vi "Synchronized PUT Channel.vi"(1 "PUT Value":string, 2 "PUT VI Reference":refnum<vi>) -> ()   [LabVIEW 2013]
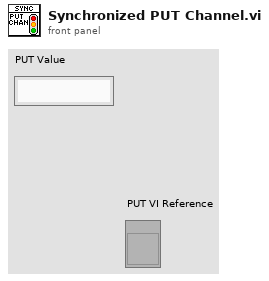
[diagram p1: front panel]
types:
  T1 = typedef "Semaphore RefNum" = refnum<k1>
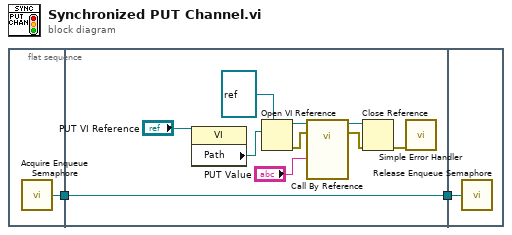
[diagram p0: block diagram]
diagram:
  n1 = flat-sequence {
    tunnel: [w3] -> w2
    tunnel: w2 -> [w13]
    tunnel: [w13] -> w1
    tunnel: w1 -> [w14]
    frame #0 {
      n2 = call "Acquire Enqueue Semaphore.vi"() -> ("Semaphore Reference"=w3:T1)
    }
    frame #1 {
      n3 = property class="VI"(reference="PUT VI Reference") -> ("Path"=w10:path)  [unwired: 1 in, 2 out]
      n4 = Open VI Reference(type specifier VI Refnum (for type only)=refnum<vi> refnum, vi path=w10) -> (vi reference=w9:refnum<vi>, error out=w8:errorcluster)  [unwired: 4 in]
      n5 = call-by-ref "?"(reference=w9, error in=w8, "X Input Channel"="PUT Value") -> (reference out=w7:refnum<vi>, error out=w6:errorcluster)
      n6 = Close Reference(reference=w7, error in (no error)=w6) -> (error out=w5:errorcluster)
      n7 = call <vilib>:"Simple Error Handler.vi"("error in (no error)"=w5) -> ()  [unwired: 4 in, 5 out]
    }
    frame #2 {
      n8 = call "Release Enqueue Semaphore.vi"("Semaphore Reference"=w14) -> ()
    }
  }
